vi "Cancel.vi"(8 "error in (no error)":errorcluster, 11 "Notifier in":refnum<class "Notifier.lvclass">) -> (0 "error out":errorcluster, 2 "Data Notification":refnum<class "Data.lvclass">, 3 "Notifier out":refnum<class "Notifier.lvclass">)   [LabVIEW 2020, in "Data.lvlib" / "Notifier.lvclass"]
doc: "Cancel the notification."
uses:
  Notifier.lvclass
  Data.lvclass
  Notifier.lvclass/Notifier.ctl
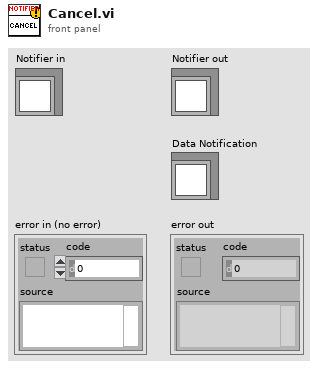
[diagram p1: front panel]
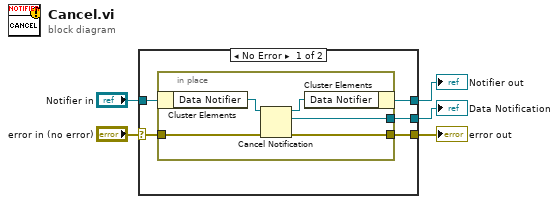
[diagram p0: block diagram]
diagram:
  n1 = case shown="No Error" "error in (no error)" {
    selector: "error in (no error)" -> [w8 w17]
    tunnel: [w7 w17] -> w4
    tunnel: [w9 w16] -> w2
    tunnel: "Notifier in" -> [w10 w16]
    tunnel: [w6 _] -> w1
    frame No Error {
      n2 = in-place {
        in-place-border: w8 -> [w11]
        in-place-border: [w13] -> w7
        in-place-border: [w12] -> w6
        n3 = in-place-cluster #1(w10) -> ("Data Notifier"=w15:refnum<notifier>)
        n4 = Cancel Notification(0:w15, 3:w11) -> (8:w14:refnum<notifier>, 9:w12:refnum<class "Data.lvclass">, 11:w13:errorcluster)
        n5 = in-place-cluster #1("Data Notifier"=w14) -> (w9:refnum<class "Notifier.lvclass">)
      }
    }
    frame Error {
    }
  }
  "error out" <- w4
  "Notifier out" <- w2
  "Data Notification" <- w1
